vi "Add Event Structure Frame.vi"(7 "After? (T)":bool, 8 "error in (no error)":errorcluster, 10 "Reference Frame Index":u32, 11 "Event Structure ref in":refnum<vi>) -> (0 "error out":errorcluster, 1 "Added Frame":refnum<vi>, 2 "Added Frame Index":i32, 3 "Event Structure ref out":refnum<vi>)   [LabVIEW 2019, in "gRPC Template Creation Utility.lvlib"]
uses:
  gRPC Template Creation Utility.lvlib
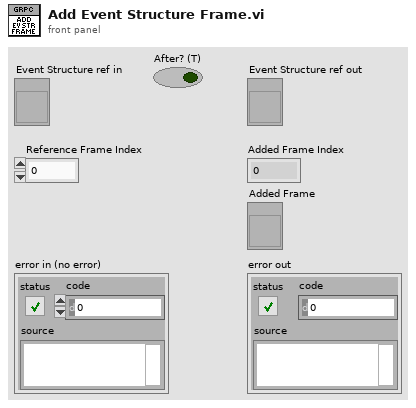
[diagram p1: front panel]
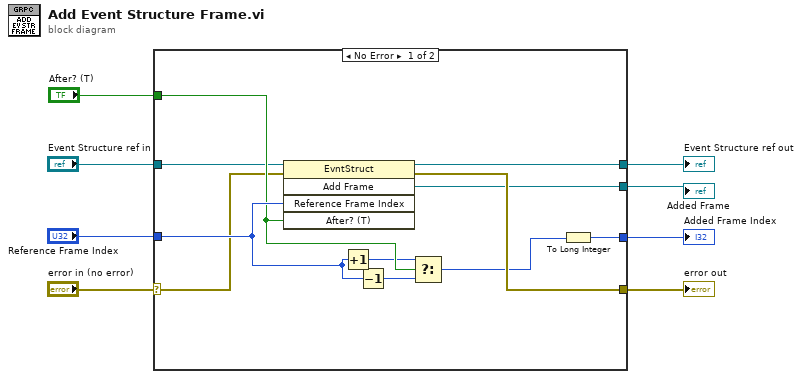
[diagram p0: block diagram]
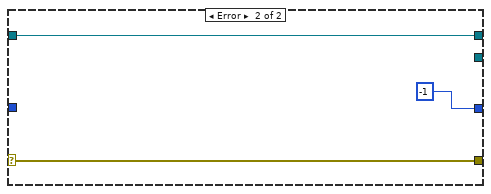
[diagram p2: hidden frame]
diagram:
  n1 = case shown="No Error" "error in (no error)" {
    selector: "error in (no error)" -> [w12 w22]
    tunnel: [w11 -1] -> w8
    tunnel: "Reference Frame Index" -> [w19 _]
    tunnel: "After? (T)" -> [w18 _]
    tunnel: [w15 w22] -> w5
    tunnel: [w14 w21] -> w4
    tunnel: "Event Structure ref in" -> [w13 w21]
    tunnel: [w9 _] -> w1
    frame No Error {
      n2 = invoke class="EvntStruct" method="Add Frame"(reference=w13, error in=w12, "Reference Frame Index"=w19, "After? (T)"=w18) -> (reference out=w14:refnum<vi>, error out=w15:errorcluster, "Add Frame"=w9:refnum<vi>)  [unwired: 1 in, 2 out]
      n3 = Increment(x=w19) -> (x+1=w16:u32)
      n4 = Decrement(x=w19) -> (x-1=w17:u32)
      n5 = Select(t=w16, s=w18, f=w17) -> (s? t:f=w10:u32)
      n6 = To Long Integer(number=w10) -> (32bit integer=w11:i32)
    }
    frame Error {
    }
  }
  "Added Frame Index" <- w8
  "error out" <- w5
  "Event Structure ref out" <- w4
  "Added Frame" <- w1
